vi "Set notifier.vi"(8 "error in (no error)":errorcluster caption="entrée d'erreur (pas d'erreur)", 10 "notifier":refnum<notifier>, 11 "Message en entrée":refnum<class "Message.lvclass">) -> (0 "error out":errorcluster caption="sortie d'erreur", 3 "Message en sortie":refnum<class "Message.lvclass">)   [LabVIEW 2020, in "Message.lvclass"]
uses:
  Message.lvclass
  Message.lvclass/Message.ctl
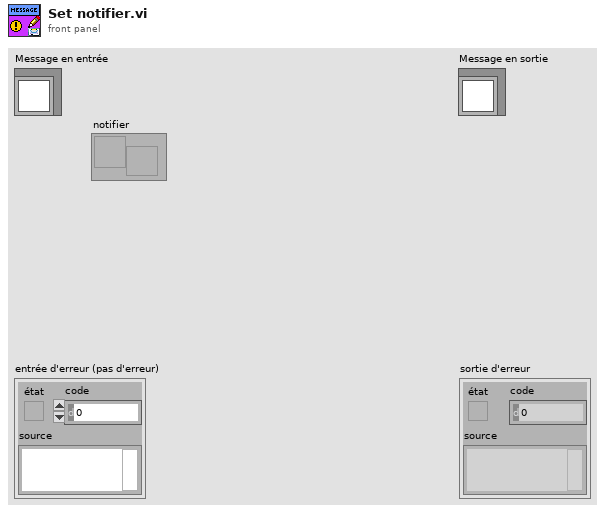
[diagram p1: front panel]
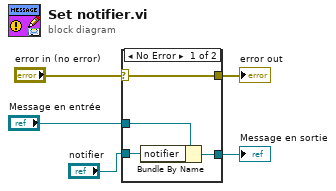
[diagram p0: block diagram]
diagram:
  n1 = case shown="No Error" "error in (no error)" {
    selector: "error in (no error)" -> [w9 w10]
    tunnel: [w9 w10] -> w4
    tunnel: [w7 w11] -> w2
    tunnel: "Message en entrée" -> [w8 w11]
    tunnel: "notifier" -> [w6 _]
    frame No Error {
      n2 = Bundle By Name(cluster=w8, "notifier"=w6) -> (w7:refnum<class "Message.lvclass">)
    }
    frame Error {
    }
  }
  "error out" <- w4
  "Message en sortie" <- w2
